vi "Memory Graph.vi"() -> ()   [LabVIEW 2020]
uses:
  <vilib>/Analysis/NI_AALBase.lvlib
panel:
  in  "stop":bool
  out "Intensity Graph":u8[][](graph)
  # "Christian Altenbach 2005, caltenba@ucla.edu"
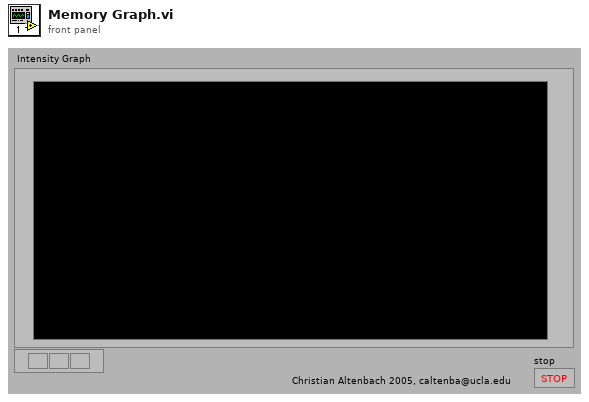
[diagram p1: front panel]
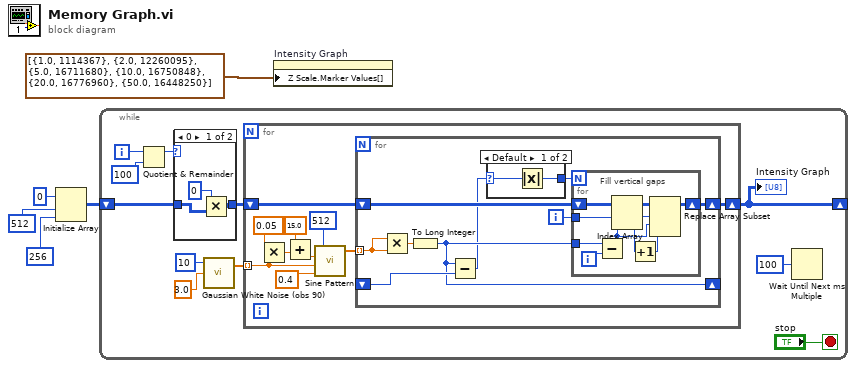
[diagram p0: block diagram]
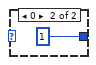
[diagram p3: hidden frame]
diagram:
  n1 = Initialize Array(u8 0 ("element"), 512 ("dimension size"), 256 ("dimension size")) -> (w5:u8[][])
  n2 = while {
    shift-right: [w12] -> _
    shift-left: w5 -> [w16]
    i -> [w8]
    stop <- "stop" stop-if-true
    n3 = Quotient & Remainder(x=w8, y=100) -> (x-y*floor(x/y)=w6:i32)  [unwired: 1 out]
    n4 = case shown="0" w6 {
      tunnel: w16 -> [w19 w20]
      tunnel: [w18 w20] -> w11
      frame 0 {
        n5 = Multiply(x=u8 0 ("standard deviation"), y=w19) -> (x*y=w18:u8[][])
      }
      frame 1, Default {
      }
    }
    n6 = call <vilib>:"Gaussian White Noise (obs 90).vi"("standard deviation"=3.0, "samples"=10) -> ("Gaussian noise pattern"=w14:dbl[])  [unwired: 1 in, 1 out]
    n7 = for {
      shift-right: [w28] -> w12
      shift-left: w11 -> [w29]
      tunnel: w14 -> [w23] mode=indexing
      n8 = Multiply(x=0.05, y=w23) -> (x*y=w22:dbl)
      n9 = Add(x=15.0 ("amplitude"), y=w22) -> (x+y=w24:dbl)
      n10 = call <vilib>:"Sine Pattern.vi"("cycles"=0.4 ("x"), "phase(degrees)"=w23, "amplitude"=w24, "samples"=512) -> ("Sinusoidal Pattern"=w26:dbl[])  [unwired: 1 out]
      n11 = for {
        shift-right: [w39] -> w28
        shift-left: w29 -> [w36]
        tunnel: w26 -> [w35] mode=indexing
        shift-right: [w34] -> _
        shift-left: _ -> [w37]
        i -> [w38]
        n12 = Multiply(x=w35, y=w35) -> (x*y=w31:dbl)
        n13 = To Long Integer(number=w31) -> (32bit integer=w34:i32)
        n14 = Subtract(x=w34, y=w37) -> (x-y=w33:i32)
        n15 = case shown="Default" w33 {
          selector: w33 -> [w40 _]
          tunnel: [w41 1] -> w32
          frame Default {
            n16 = Absolute Value(x=w40) -> (abs(x)=w41:i32)
          }
          frame 0 {
          }
        }
        n17 = for {
          N: w32 -> [_]
          tunnel: w38 -> [w46]
          shift-right: [w50] -> w39
          shift-left: w36 -> [w47]
          tunnel: w34 -> [w43]
          i -> [w44]
          # "Fill vertical gaps"
          n18 = Subtract(x=w43, y=w44) -> (x-y=w45:i32)
          n19 = Index Array(array=w47, index (row)=w46, index (col)=w45) -> (element=w48:u8)
          n20 = Increment(x=w48) -> (x+1=w49:u8)
          n21 = Replace Array Subset(array=w47, new element=w49, index (row)=w46, index (col)=w45) -> (w50:u8[][])
        }
      }
    }
    "Intensity Graph" <- w12
    n22 = Wait Until Next ms Multiple(millisecond multiple=u32 100) -> ()  [unwired: 1 out]
  }
  n23 = property on="Intensity Graph" class="IntGraph (strict)"("Z Scale.Marker Values[]"=cluster{dbl, u32}[] [{1.0, 1114367}, {2.0, 12260095}, {5.0, 16711680}, {10.0, 16750848}, {20.0, 16776960}, {50.0, 16448250}]) -> ()  [unwired: 2 in, 2 out]
